vi "4.1.vi"() -> ()   [LabVIEW 2017]
panel:
  out "Waveform Graph 2":dynamicdata(graph)
  out "Waveform Graph":dynamicdata(graph)
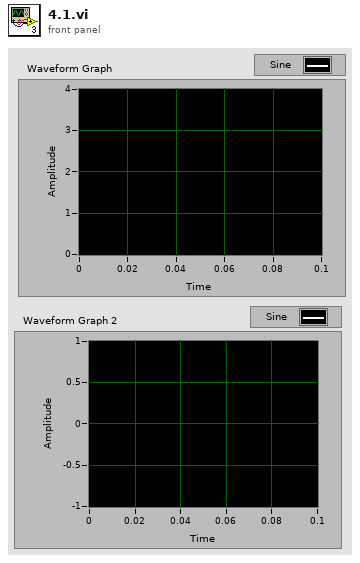
[diagram p1: front panel]
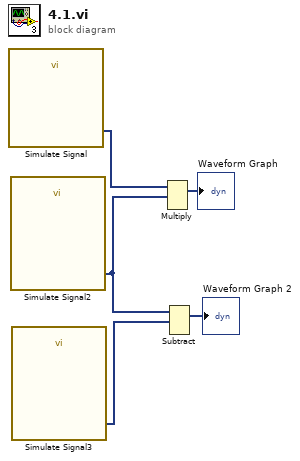
[diagram p0: block diagram]
diagram:
  n1 = call "Simulate Signal"() -> ("Sine"=w5:dynamicdata)  [unwired: 14 in, 1 out]
  n2 = call "Simulate Signal2"() -> ("Sine"=w4:dynamicdata)  [unwired: 14 in, 1 out]
  n3 = call "Simulate Signal3"() -> ("Sine"=w3:dynamicdata)  [unwired: 14 in, 1 out]
  n4 = Multiply(1:w4, 2:w5) -> (0:→"Waveform Graph":dynamicdata)  [unwired: 1 in, 1 out]
  n5 = Subtract(1:w3, 2:w4) -> (0:→"Waveform Graph 2":dynamicdata)  [unwired: 1 in, 1 out]
